vi "HEWH Power Cluster Calcs.vi"(0 "Voltage":dbl=240.0, 5 "Watts":dbl, 7 "WattHours":dbl) -> (6 "PowerData":T1={"Voltage"=240.0, "Current"=0.017575, "Power"=4.218, "WattHours"=19682.0}, 8 "PowerClass":T2={"Off"=FALSE, "On"=TRUE, "Fans"=FALSE, "Compressor"=FALSE, "Heat Elem."=TRUE, "Fault-OverPwr"=FALSE})   [LabVIEW 2012]
uses:
  PowerClassification.ctl
  PowerData.ctl
panel:
  in  "FanLL":dbl=0.01
  in  "Fault Limit":dbl=5000.0
  in  "CompressorUL":dbl=2.0
  in  "CompressorLL":dbl=0.3
  in  "Off Limit":dbl=0.001
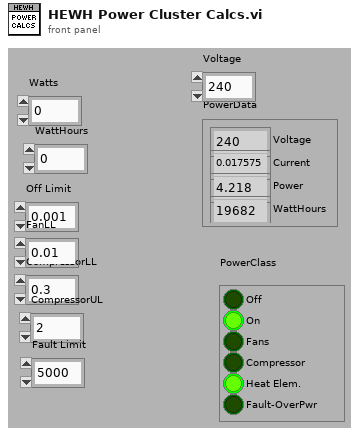
[diagram p1: front panel]
types:
  T1 = typedef "PowerData.ctl" = cluster{"Voltage":dbl, "Current":dbl, "Power":dbl, "WattHours":dbl}
  T2 = typedef "PowerClassification.ctl" = cluster{"Off":bool, "On":bool, "Fans":bool, "Compressor":bool, "Heat Elem.":bool, "Fault-OverPwr":bool}
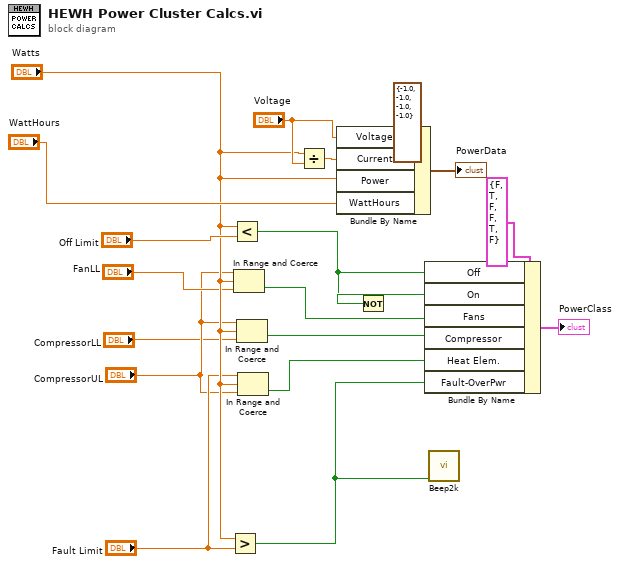
[diagram p0: block diagram]
diagram:
  n1 = Greater?(x="Watts", y="Fault Limit") -> (0:w7:bool)
  n2 = Less?(x="Watts", y="Off Limit") -> (x < y?=w18:bool)
  n3 = In Range and Coerce(upper limit="CompressorUL", x="Watts", lower limit="FanLL") -> (In Range?=w4:bool)  [unwired: 1 out]
  n4 = In Range and Coerce(upper limit="CompressorUL", x="Watts", lower limit="CompressorLL") -> (In Range?=w6:bool)  [unwired: 1 out]
  n5 = In Range and Coerce(upper limit="Fault Limit", x="Watts", lower limit="CompressorUL") -> (In Range?=w16:bool)  [unwired: 1 out]
  n6 = Divide(x="Watts", y="Voltage") -> (x/y=w11:dbl)
  n7 = Bundle By Name(cluster=T1 {"Voltage"=-1.0, "Current"=-1.0, "Power"=-1.0, "WattHours"=-1.0} ("PowerData"), "Voltage"="Voltage", "Current"=w11, "Power"="Watts", "WattHours"="WattHours") -> (→"PowerData":T1)
  n8 = Not(x=w18) -> (.not. x?=w19:bool)
  n9 = Bundle By Name(cluster=T2 {"Off"=FALSE, "On"=TRUE, "Fans"=FALSE, "Compressor"=FALSE, "Heat Elem."=TRUE, "Fault-OverPwr"=FALSE} ("PowerClass 2"), "Off"=w18, "On"=w19, "Fans"=w4, "Compressor"=w6, "Heat Elem."=w16, "Fault-OverPwr"=w7) -> (→"PowerClass":T2)
  n10 = call "Beep2k.vi"("Beep?"=w7) -> ()  [unwired: 11 in]
